vi "RepIntOut.vi"(8 "output cluster":T1, 11 "Diff Index":dbl) -> (3 "Output":dbl)   [LabVIEW 2010, in "KevLib01.lvlib"]
uses:
  KevLib01.lvlib
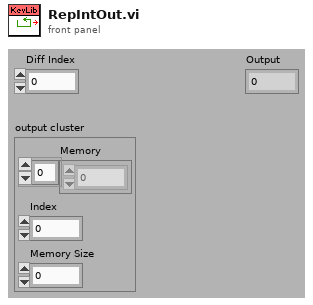
[diagram p1: front panel]
types:
  T1 = cluster{"Memory":dbl[], "Index":i32, "Memory Size":i32}
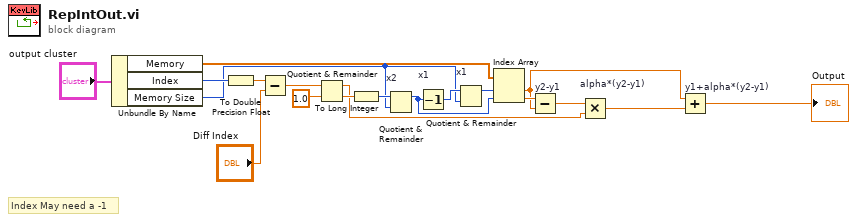
[diagram p0: block diagram]
diagram:
  # "Index May need a -1"
  n1 = Unbundle By Name("output cluster") -> ("Memory"=w14:dbl[], "Index"=w10:i32, "Memory Size"=w2:i32)
  n2 = To Double Precision Float(number=w10) -> (double precision float=w9:dbl)
  n3 = Subtract(x=w9, y="Diff Index") -> (x-y=w1:dbl)
  n4 = Quotient & Remainder(x=w1, y=1.0) -> (x-y*floor(x/y)=w3:dbl, floor(x/y)=w13:dbl)
  n5 = To Long Integer(number=w13) -> (32bit integer=w7:i32)
  n6 = Quotient & Remainder "x2"(x=w7, y=w2) -> (x-y*floor(x/y)=w17:i32)  [unwired: 1 out]
  n7 = Decrement "x1"(x=w17) -> (x-1=w15:i32)
  n8 = Quotient & Remainder "x1"(x=w15, y=w2) -> (x-y*floor(x/y)=w16:i32)  [unwired: 1 out]
  n9 = Index Array(array=w14, index #1=w16, index #2=w17) -> (element #1=w5:dbl, element #2=w18:dbl)
  n10 = Subtract "y2-y1"(x=w18, y=w5) -> (x-y=w19:dbl)
  n11 = Multiply "alpha*(y2-y1)"(x=w19, y=w3) -> (x*y=w6:dbl)
  n12 = Add "y1+alpha*(y2-y1)"(x=w5, y=w6) -> (x+y=→"Output":dbl)
